vi "test Comparison.vi"(8 "error in (no error)":errorcluster, 11 "Dummy In":refnum<class "Dummy.lvclass">) -> (0 "error out":errorcluster, 3 "Dummy Out":refnum<class "Dummy.lvclass">)   [LabVIEW 2020, in "Dummy.lvclass"]
doc: "Test case with comparison"
uses:
  Dummy.lvclass
  C:/git/astemes-lunit/source/API/LUnit Test Case/LUnit Test Case.lvclass
  API/LUnit Test Case/LUnit Test Case.lvclass/LUnit Test Case.ctl
  b9db8760-c0fc-4f58-bd52-c7853f173bcb.vi
  c67ca9b7-f05b-4050-9a64-1f171d30ec2c.vi
  da6a2475-a5ba-4c24-a32d-a20b797c7be8.vi
  39c04321-5979-4a3e-a701-3af7a453472c.vi
  0e564e09-6605-4779-ac5a-7c25b3aad5a0.vi
  API/LUnit Test Case/Private/Append Pass Result.vi
  API/LUnit Test Case/Private/Append Fail Result.vi
  API/LUnit Test Case/Private/Compare Variants.vi
  API/LUnit Test Case/Private/Describe Comparison.vi
  API/LUnit Test Case/Private/Variant to string.vi
  <vilib>/Utility/Data Type/Get Type Information.vi
  <vilib>/Utility/LVClass/Get LV Class Name.vi
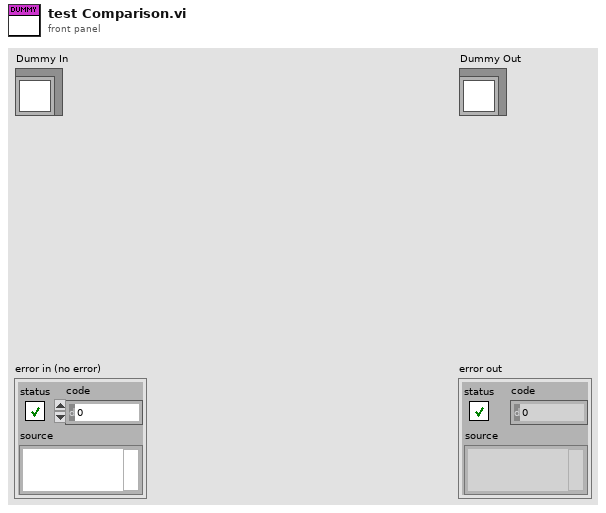
[diagram p1: front panel]
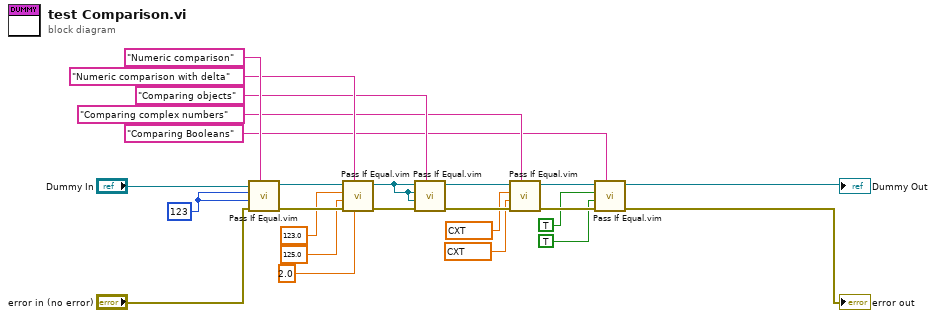
[diagram p0: block diagram]
diagram:
  w23 = 123
  n1 = call "Pass If Equal.vim"("Description"="Numeric comparison", "error in (no error)"="error in (no error)", "Actual"=w23, "Expected"=w23, "LUnit Test Case In"="Dummy In") -> ("error out"=w20:errorcluster, "LUnit Test Case Out"=w21:refnum<class "Dummy.lvclass">)  [unwired: 5 in]
  n2 = call "Pass If Equal.vim"("Delta"=2.0, "Description"="Numeric comparison with delta", "error in (no error)"=w20, "Actual"=125.0, "Expected"=123.0, "LUnit Test Case In"=w21) -> ("error out"=w15:errorcluster, "LUnit Test Case Out"=w14:refnum<class "Dummy.lvclass">)  [unwired: 4 in]
  n3 = call "Pass If Equal.vim"("Description"="Comparing objects", "error in (no error)"=w15, "Actual"=w14, "Expected"=w14, "LUnit Test Case In"=w14) -> ("error out"=w11:errorcluster, "LUnit Test Case Out"=w12:refnum<class "Dummy.lvclass">)  [unwired: 5 in]
  n4 = call "Pass If Equal.vim"("Description"="Comparing complex numbers", "error in (no error)"=w11, "Actual"=cxt 123.0+0.0i, "Expected"=cxt 123.0+0.0i, "LUnit Test Case In"=w12) -> ("error out"=w6:errorcluster, "LUnit Test Case Out"=w7:refnum<class "Dummy.lvclass">)  [unwired: 5 in]
  n5 = call "Pass If Equal.vim"("Description"="Comparing Booleans", "error in (no error)"=w6, "Actual"=TRUE, "Expected"=TRUE, "LUnit Test Case In"=w7) -> ("error out"=→"error out":errorcluster, "LUnit Test Case Out"=→"Dummy Out":refnum<class "Dummy.lvclass">)  [unwired: 5 in]
